vi "LJM make factory settings config files.vi"(3 "Working Directory":path) -> ()   [LabVIEW 2025]
uses:
  LJstreamM globals.vi
  <vilib>/Utility/config.llb/Write Key (String).vi
  <vilib>/Utility/config.llb/Write Key (U32).vi
  <vilib>/Utility/config.llb/Write Key (Double).vi
  <vilib>/Utility/config.llb/Write Key (I32).vi
  <vilib>/Utility/config.llb/Write Key (Boolean).vi
  <vilib>/Utility/config.llb/NI_LVConfig.lvlib
panel:
  out "error out 2":errorcluster
  out "error out":errorcluster
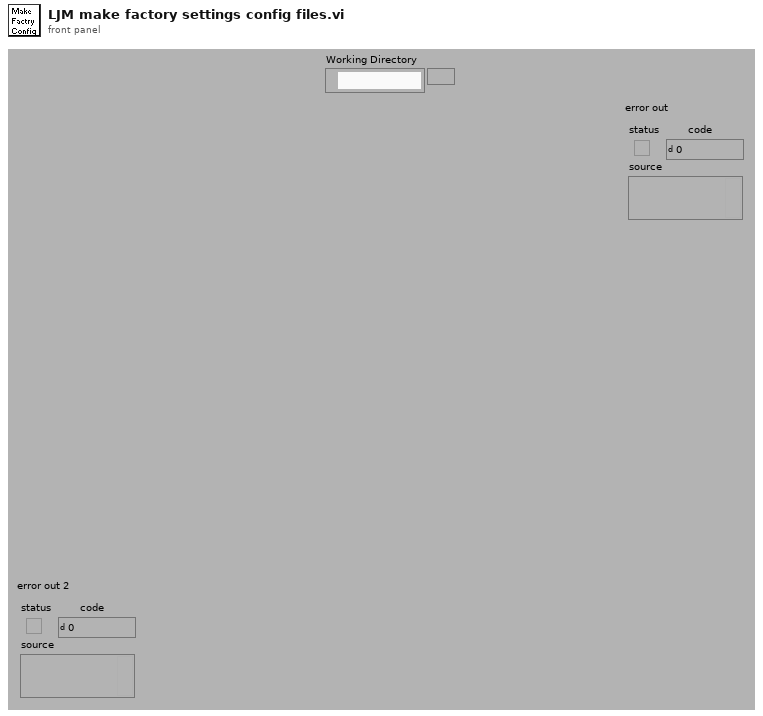
[diagram p1: front panel]
types:
  T1 = typedef "NI_LVConfig.lvlib/Config Data RefNum.ctl" = refnum<k1>
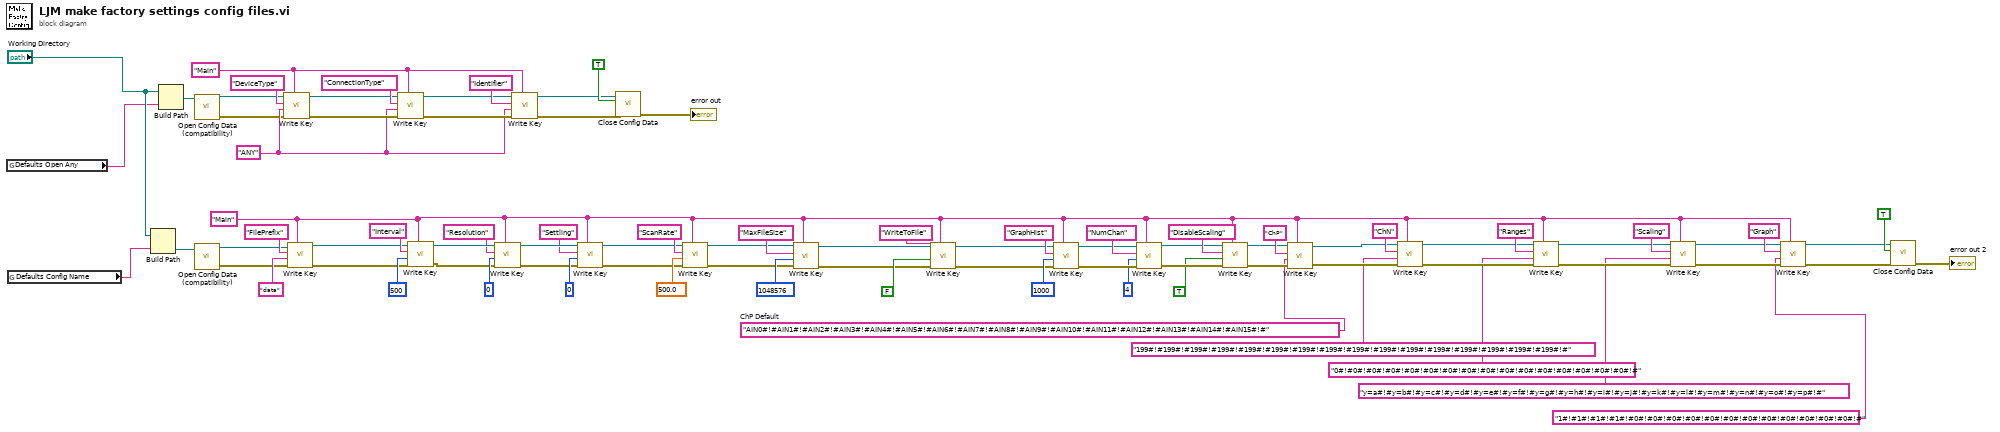
[diagram p0: block diagram]
diagram:
  w4 = "AIN0#!#AIN1#!#AIN2#!#AIN3#!#AIN4#!#AIN5#!#AIN6#!#AIN7#!#AIN8#!#AIN9#!#AIN10#!#AIN11#!#AIN12#!#AIN13#!#AIN14#!#AIN15#!#"  # ChP Default
  w10 = "Main" ("section")
  w72 = "ANY" ("Data File Prefix")
  w73 = "Main" ("section")
  n1 = global read "LJstreamM globals.vi" "Defaults Open Any"() -> (w1:string)
  n2 = global read "LJstreamM globals.vi" "Defaults Config Name"() -> (w2:string)
  n3 = Build Path(base path="Working Directory", name or relative path=w2) -> (appended path=w70:path)
  n4 = Build Path(base path="Working Directory", name or relative path=w1) -> (appended path=w75:path)
  n5 = call <vilib>:"Open Config Data (compatibility).vi"("configuration file path"=w75) -> ("error out"=w5:errorcluster, "refnum"=w6:T1)  [unwired: 8 in, 1 out]
  n6 = call <vilib>:"Open Config Data (compatibility).vi"("configuration file path"=w70) -> ("error out"=w8:errorcluster, "refnum"=w9:T1)  [unwired: 8 in, 1 out]
  n7 = call-poly <vilib>:"Write Key.vi"("section"=w73, "error in (no error)"=w5, "value"=w72, "key"="DeviceType", "refnum"=w6) -> ("error out"=w81:errorcluster, "refnum out"=w80:T1)  [unwired: 4 in, 1 out]
  n8 = call-poly <vilib>:"Write Key.vi"("section"=w10, "error in (no error)"=w8, "value"="data" ("Data File Prefix"), "key"="FilePrefix", "refnum"=w9) -> ("error out"=w25:errorcluster, "refnum out"=w23:T1)  [unwired: 4 in, 1 out]
  n9 = call-poly <vilib>:"Write Key.vi"("section"=w73, "error in (no error)"=w81, "value"=w72, "key"="ConnectionType", "refnum"=w80) -> ("error out"=w79:errorcluster, "refnum out"=w78:T1)  [unwired: 4 in, 1 out]
  n10 = call-poly <vilib>:"Write Key.vi"("section"=w10, "error in (no error)"=w25, "value"=u32 500 ("Scan Rate (Hz)"), "key"="Interval", "refnum"=w23) -> ("error out"=w30:errorcluster, "refnum out"=w29:T1)  [unwired: 4 in, 1 out]
  n11 = call-poly <vilib>:"Write Key.vi"("section"=w10, "error in (no error)"=w30, "value"=u8 0 ("Graph History"), "key"="Resolution", "refnum"=w29) -> ("error out"=w32:errorcluster, "refnum out"=w31:T1)  [unwired: 4 in, 1 out]
  n12 = call-poly <vilib>:"Write Key.vi"("section"=w73, "error in (no error)"=w79, "value"=w72, "key"="Identifier", "refnum"=w78) -> ("error out"=w76:errorcluster, "refnum out"=w77:T1)  [unwired: 4 in, 1 out]
  n13 = call-poly <vilib>:"Write Key.vi"("section"=w10, "error in (no error)"=w32, "value"=u8 0 ("# Channels"), "key"="Settling", "refnum"=w31) -> ("error out"=w24:errorcluster, "refnum out"=w22:T1)  [unwired: 4 in, 1 out]
  n14 = call <vilib>:"Close Config Data.vi"("error in (no error)"=w76, "write file if changed (T)"=TRUE ("write configuration file? (F)"), "refnum"=w77) -> ("error out"=→"error out":errorcluster)  [unwired: 7 in, 1 out]
  n15 = call-poly <vilib>:"Write Key.vi"("section"=w10, "error in (no error)"=w24, "value"=500.0 ("Scan Rate (Hz)"), "key"="ScanRate", "refnum"=w22) -> ("error out"=w18:errorcluster, "refnum out"=w17:T1)  [unwired: 4 in, 1 out]
  n16 = call-poly <vilib>:"Write Key.vi"("section"=w10, "error in (no error)"=w18, "value"=1048576 ("Graph History"), "key"="MaxFileSize", "refnum"=w17) -> ("error out"=w13:errorcluster, "refnum out"=w14:T1)  [unwired: 4 in, 1 out]
  n17 = call-poly <vilib>:"Write Key.vi"("section"=w10, "error in (no error)"=w13, "value"=FALSE ("default value"), "key"="WriteToFile", "refnum"=w14) -> ("error out"=w11:errorcluster, "refnum out"=w12:T1)  [unwired: 4 in, 1 out]
  n18 = call-poly <vilib>:"Write Key.vi"("section"=w10, "error in (no error)"=w11, "value"=1000 ("Graph History"), "key"="GraphHist", "refnum"=w12) -> ("error out"=w65:errorcluster, "refnum out"=w66:T1)  [unwired: 4 in, 1 out]
  n19 = call-poly <vilib>:"Write Key.vi"("section"=w10, "error in (no error)"=w65, "value"=4 ("# Channels"), "key"="NumChan", "refnum"=w66) -> ("error out"=w44:errorcluster, "refnum out"=w45:T1)  [unwired: 4 in, 1 out]
  n20 = call-poly <vilib>:"Write Key.vi"("section"=w10, "error in (no error)"=w44, "value"=TRUE ("default value"), "key"="DisableScaling", "refnum"=w45) -> ("error out"=w42:errorcluster, "refnum out"=w41:T1)  [unwired: 4 in, 1 out]
  n21 = call-poly <vilib>:"Write Key.vi"("section"=w10, "error in (no error)"=w42, "value"=w4, "key"="ChP", "refnum"=w41) -> ("error out"=w60:errorcluster, "refnum out"=w61:T1)  [unwired: 4 in, 1 out]
  n22 = call-poly <vilib>:"Write Key.vi"("section"=w10, "error in (no error)"=w60, "value"="199#!#199#!#199#!#199#!#199#!#199#!#199#!#199#!#199#!#199#!#199#!#199#!#199#!#199#!#199#!#199#!#" ("Data File Prefix"), "key"="ChN", "refnum"=w61) -> ("error out"=w59:errorcluster, "refnum out"=w58:T1)  [unwired: 4 in, 1 out]
  n23 = call-poly <vilib>:"Write Key.vi"("section"=w10, "error in (no error)"=w59, "value"="0#!#0#!#0#!#0#!#0#!#0#!#0#!#0#!#0#!#0#!#0#!#0#!#0#!#0#!#0#!#0#!#" ("Data File Prefix"), "key"="Ranges", "refnum"=w58) -> ("error out"=w56:errorcluster, "refnum out"=w55:T1)  [unwired: 4 in, 1 out]
  n24 = call-poly <vilib>:"Write Key.vi"("section"=w10, "error in (no error)"=w56, "value"="y=a#!#y=b#!#y=c#!#y=d#!#y=e#!#y=f#!#y=g#!#y=h#!#y=i#!#y=j#!#y=k#!#y=l#!#y=m#!#y=n#!#y=o#!#y=p#!#" ("Data File Prefix"), "key"="Scaling", "refnum"=w55) -> ("error out"=w39:errorcluster, "refnum out"=w36:T1)  [unwired: 4 in, 1 out]
  n25 = call-poly <vilib>:"Write Key.vi"("section"=w10, "error in (no error)"=w39, "value"="1#!#1#!#1#!#1#!#0#!#0#!#0#!#0#!#0#!#0#!#0#!#0#!#0#!#0#!#0#!#0#!#" ("Data File Prefix"), "key"="Graph", "refnum"=w36) -> ("error out"=w38:errorcluster, "refnum out"=w37:T1)  [unwired: 4 in, 1 out]
  n26 = call <vilib>:"Close Config Data.vi"("error in (no error)"=w38, "write file if changed (T)"=TRUE ("write configuration file? (F)"), "refnum"=w37) -> ("error out"=→"error out 2":errorcluster)  [unwired: 7 in, 1 out]
